vi "SonarRead.vi"(10 "Sonar Number":enum16{"Sonar 0", "Sonar 1", "Sonar 2"}(ring), 11 "FPGA VI Reference In":refnum<k20>) -> (2 "Sonar Reading":i32, 3 "FPGA VI Reference Out":refnum<k20>)   [LabVIEW 2013]
uses:
  <vilib>/rvi/interface/common/niFpgaWaitOnOcc.vi
  <vilib>/Utility/error.llb/Error Cluster From Error Code.vi
  <vilib>/rvi/errors/niLvFpgaAdjustHostInterfaceError.vi
  <vilib>/rvi/interface/nirviReadWriteControl/nirviReadWriteControl.xnode
  NiFpgaLv.dll
  <vilib>/rvi/interface/Simulation/niFpgaSimulationCallBeginRW.vi
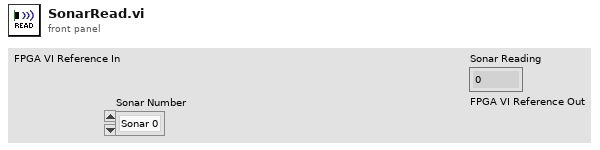
[diagram p1: front panel]
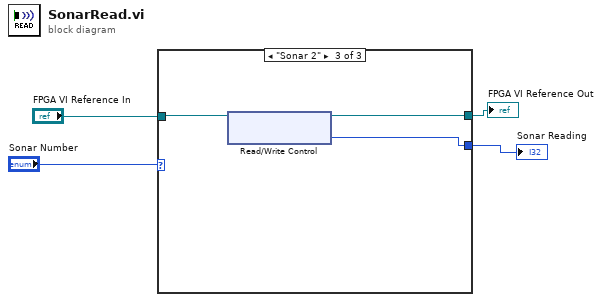
[diagram p0: block diagram]
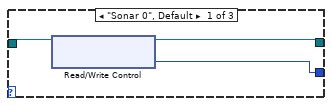
[diagram p2: hidden frame]
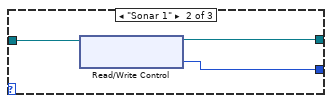
[diagram p3: hidden frame]
diagram:
  n1 = case shown="\"Sonar 2\"" "Sonar Number" {
    tunnel: "FPGA VI Reference In" -> [w7 w10 w13]
    tunnel: [w5 w9 w11] -> w3
    tunnel: [w6 w8 w12] -> w2
    frame "Sonar 0", Default {
      n2 = xnode "Read/Write Control"("FPGA VI Reference In"=w7) -> ("FPGA VI Reference Out"=w6:refnum<k20>, "Sonar Reading 0"=w5:i32)  [unwired: 1 in, 1 out]
    }
    frame "Sonar 1" {
      n3 = xnode "Read/Write Control"("FPGA VI Reference In"=w10) -> ("FPGA VI Reference Out"=w8:refnum<k20>, "Sonar Reading 1"=w9:i32)  [unwired: 1 in, 1 out]
    }
    frame "Sonar 2" {
      n4 = xnode "Read/Write Control"("FPGA VI Reference In"=w13) -> ("FPGA VI Reference Out"=w12:refnum<k20>, "Sonar Reading 2"=w11:i32)  [unwired: 1 in, 1 out]
    }
  }
  "Sonar Reading" <- w3
  "FPGA VI Reference Out" <- w2
